vi "test..vi"() -> ()   [LabVIEW 2020]
uses:
  <vilib>/Analysis/baseanly.llb/Mean (DBL).vi
  Oscilloscope/TELEDINE_LECROY/LeCroy Wave Series/LeCroy Wave Series.lvlib
  <vilib>/Analysis/NI_AALBase.lvlib
panel:
  out "Array 2":dbl[](array[numeric])
  out "Array":waveform(dbl)[](array[waveform])
  out "elyse clock":dbl format="%0.2f"
  out "lecroy":dbl format="%0.2f"
  out "error out":errorcluster
  out "max":i8[](array[numeric])
  out "elyse":i32
  out "output array":dbl[](array[numeric])
  out "Waveform Graph":waveform(dbl)(graph)
  in  "Boolean":bool
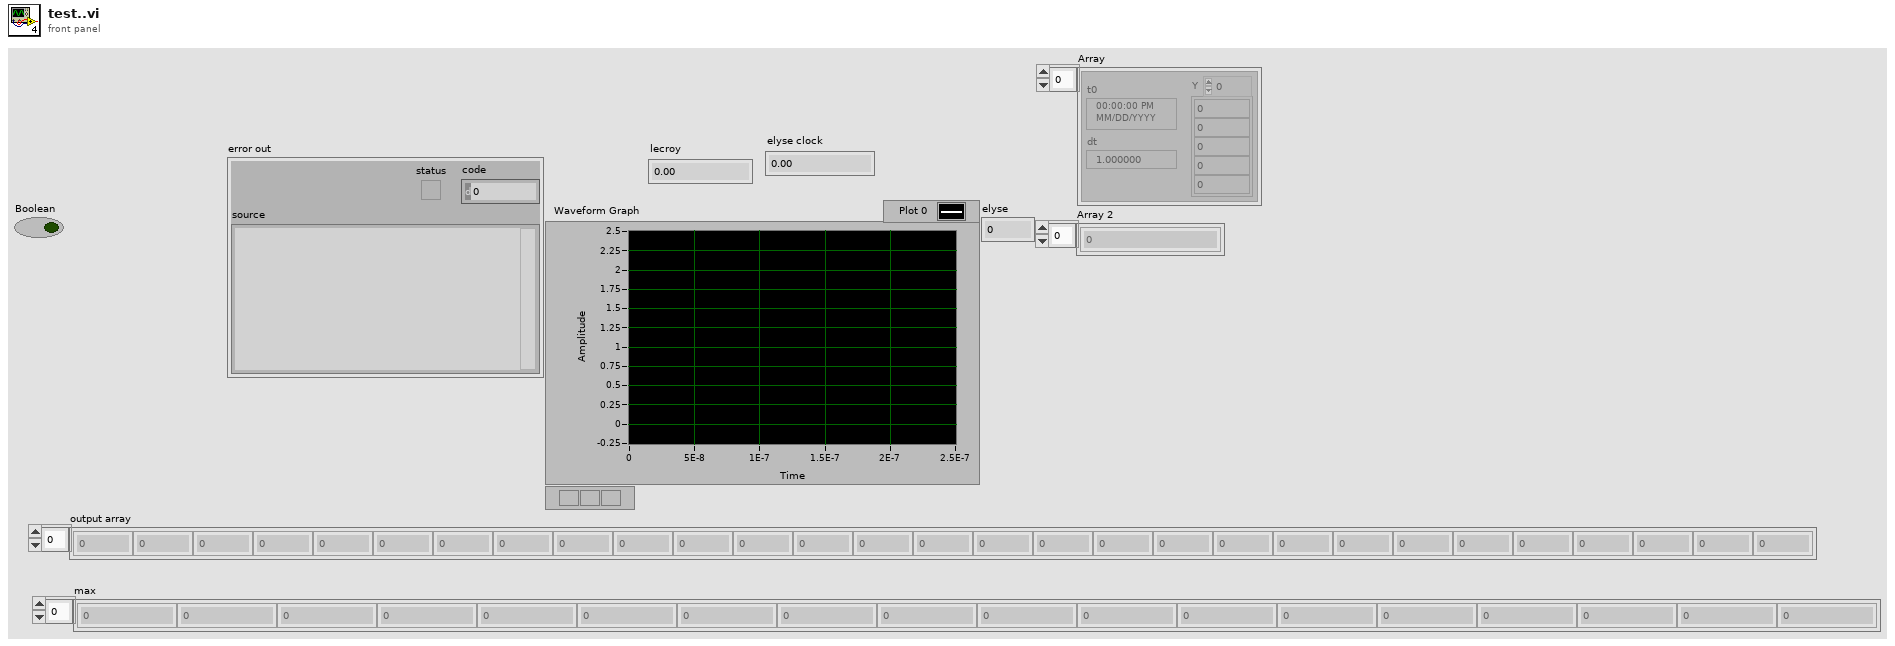
[diagram p1: front panel]
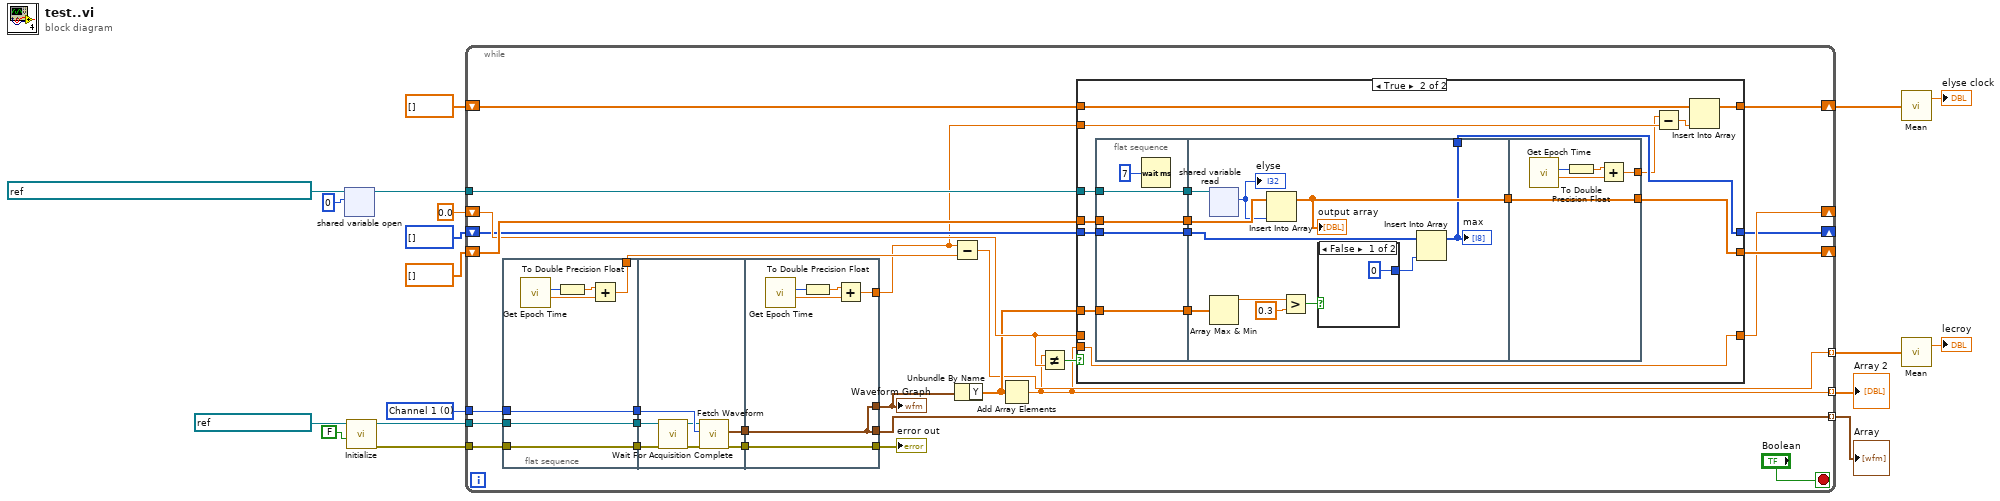
[diagram p0: block diagram]
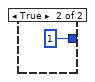
[diagram p3: hidden frame]
diagram:
  w12 = u16 0 items=["Channel 1", "Channel 2", "Channel 3", "Channel 4", "Memory 1", "Memory 2", "Memory 3", "Memory 4", "Function 1", "Function 2", "Function 3", "Function 4", "Function 5", "Function 6", "Function 7", "Function 8", "Other"] ("Source (0: Channel 1)")
  n1 = shared-variable-open(refnum<k21> "ni.var.psp://my computer/elyse_variables/elyse_counts" ("shared variable refnum in"), 0) -> (w17:refnum<k21>)  [unwired: 2 in, 1 out]
  n2 = call "Initialize.vi"("Reset? (T: Yes)"=FALSE, "VISA resource name"=refnum<visa-resource-name> "VICP::10.20.30.199") -> ("error out"=w9:errorcluster, "VISA resource name out"=w10:refnum<visa-resource-name>)  [unwired: 8 in]
  n3 = while {
    tunnel: w17 -> [w41]
    shift-right: [w44] -> _
    shift-left: dbl[] [] -> [w45]
    shift-right: [w43] -> _
    shift-left: 0.0 -> [w42]
    shift-right: [w38] -> _
    shift-left: i8[] [] -> [w39]
    tunnel: w10 -> [w37]
    tunnel: w12 -> [w36]
    tunnel: w9 -> [w34]
    tunnel: [w25] -> w7 mode=indexing
    shift-right: [w22] -> w3
    shift-left: dbl[] [] -> [w23]
    tunnel: [w20] -> w2 mode=indexing
    tunnel: [w19] -> w1 mode=indexing
    stop <- "Boolean" stop-if-true
    n4 = flat-sequence {
      tunnel: w34 -> [w94]
      tunnel: w36 -> [w95]
      tunnel: w37 -> [w96]
      tunnel: [w96] -> w31
      tunnel: [w95] -> w30
      tunnel: [w94] -> w29
      tunnel: [w90] -> w26
      tunnel: w31 -> [w100]
      tunnel: w30 -> [w103]
      tunnel: w29 -> [w97]
      tunnel: [w102] -> w28
      tunnel: [w101] -> w27
      tunnel: [w109] -> w32
      tunnel: [w104] -> w35
      tunnel: w28 -> [w104]
      tunnel: w27 -> [w109]
      tunnel: [w105] -> w24
      tunnel: [w104] -> w20
      frame #0 {
        n5 = call <vilib>:"Get Epoch Time.vi"() -> ("Fractional Second"=w93:dbl, "Epoch Time (s)"=w91:i64)  [unwired: 9 in, 1 out]
        n6 = To Double Precision Float(number=w91) -> (double precision float=w92:dbl)
        n7 = Add(x=w92, y=w93) -> (x+y=w90:dbl)
      }
      frame #1 {
        n8 = call "Wait For Acquisition Complete.vi"("error in (no error)"=w97, "VISA resource name"=w100) -> ("error out"=w98:errorcluster, "VISA resource name out"=w99:refnum<visa-resource-name>)  [unwired: 7 in, 1 out]
        n9 = call "Fetch Waveform.vi"("error in (no error)"=w98, "Source (0: Channel 1)"=w103, "VISA resource name"=w99) -> ("error out"=w101:errorcluster, "Waveform Graph"=w102:waveform(dbl))  [unwired: 6 in, 1 out]
      }
      frame #2 {
        n10 = call <vilib>:"Get Epoch Time.vi"() -> ("Fractional Second"=w106:dbl, "Epoch Time (s)"=w108:i64)  [unwired: 9 in, 1 out]
        n11 = To Double Precision Float(number=w108) -> (double precision float=w107:dbl)
        n12 = Add(x=w107, y=w106) -> (x+y=w105:dbl)
      }
    }
    n13 = Subtract(x=w24, y=w26) -> (x-y=w25:dbl)
    n14 = Unbundle By Name(w35) -> ("Y"=w33:dbl[])
    n15 = Add Array Elements(numeric array=w33) -> (sum=w19:dbl)
    n16 = Not Equal?(x=w19, y=w42) -> (x != y?=w21:bool)
    n17 = case shown="True" w21 {
      tunnel: w45 -> [w49 w66]
      tunnel: [w49 w63] -> w44
      tunnel: [w48 w65] -> w43
      tunnel: w19 -> [_ w65]
      tunnel: w42 -> [w48 _]
      tunnel: w41 -> [_ w64]
      tunnel: w39 -> [w47 w62]
      tunnel: [w47 w61] -> w38
      tunnel: w33 -> [_ w60]
      tunnel: w24 -> [_ w59]
      tunnel: w23 -> [w46 w58]
      tunnel: [w46 w57] -> w22
      frame False {
      }
      frame True {
        n18 = flat-sequence {
          tunnel: w60 -> [w68]
          tunnel: w62 -> [w69]
          tunnel: w64 -> [w70]
          tunnel: w66 -> [w71]
          tunnel: [w71] -> w53
          tunnel: [w70] -> w52
          tunnel: [w69] -> w51
          tunnel: [w68] -> w50
          tunnel: [w77] -> w61
          tunnel: [w79] -> w55
          tunnel: w53 -> [w82]
          tunnel: w52 -> [w81]
          tunnel: w51 -> [w78]
          tunnel: w50 -> [w76]
          tunnel: [w89] -> w63
          tunnel: w55 -> [w89]
          tunnel: [w85] -> w54
          frame #0 {
            n19 = Wait (ms)(milliseconds to wait=u32 7) -> ()  [unwired: 1 out]
          }
          frame #1 {
            n20 = shared-variable-read(w81) -> (w80:i32)  [unwired: 1 in, 3 out]
            "elyse" <- w80
            n21 = Array Max & Min(array=w76) -> (max value=w75:dbl)  [unwired: 3 out]
            n22 = Insert Into Array(array=w82, new element=w80) -> (w79:dbl[])  [unwired: 1 in]
            "output array" <- w79
            n23 = Greater?(x=w75, y=0.3) -> (0:w73:bool)
            n24 = case shown="False" w73 {
              tunnel: [0 1] -> w72
              frame False {
              }
              frame True {
              }
            }
            n25 = Insert Into Array(array=w78, new element=w72) -> (w77:i8[])  [unwired: 1 in]
            "max" <- w77
          }
          frame #2 {
            n26 = call <vilib>:"Get Epoch Time.vi"() -> ("Fractional Second"=w88:dbl, "Epoch Time (s)"=w86:i64)  [unwired: 9 in, 1 out]
            n27 = To Double Precision Float(number=w86) -> (double precision float=w87:dbl)
            n28 = Add(x=w87, y=w88) -> (x+y=w85:dbl)
          }
        }
        n29 = Subtract(x=w54, y=w59) -> (x-y=w56:dbl)
        n30 = Insert Into Array(array=w58, new element=w56) -> (w57:dbl[])  [unwired: 1 in]
      }
    }
    "Waveform Graph" <- w35
    "error out" <- w32
  }
  "Array" <- w2
  "Array 2" <- w1
  n31 = call-poly <vilib>:"Mean.vi"("X"=w3) -> ("mean"=→"elyse clock":dbl)  [unwired: 1 out]
  n32 = call-poly <vilib>:"Mean.vi"("X"=w7) -> ("mean"=→"lecroy":dbl)  [unwired: 1 out]
